vi "FPGA_main_IOtest_v2.vi"() -> ()   [LabVIEW 2020]
doc: "AI and AO only for the required channels, named"
uses:
  Components/FPGA TypeDefs/SelectExcitation_Enum.ctl
  Components/FPGA TypeDefs/SelectAOchannel_Enum.ctl
  <vilib>/Platform/TimedLoop/XDataNode/timing_clust.ctl
  <vilib>/Platform/TimedLoop/XDataNode/nitl_modes.ctl
  <vilib>/Platform/TimedLoop/XDataNode/wakeup.ctl
  <vilib>/rvi/Emulation/niFpgaGetClockAttributes.vi
  <vilib>/rvi/Emulation/niFpgaSctlEmulationGetInTimedLoop.vi
  <vilib>/rvi/Emulation/niFpgaEmulationReportErrorSimple.vi
  <vilib>/rvi/eio/common/nirviEmuTemplateMethod_errors.vi
  <vilib>/rvi/Emulation/niFpgaEmulationIsFPGAContextNoSignature.vi
  <vilib>/rvi/errors/niFpgaSetErrorForExecOnDevCompSimple.vi
  <vilib>/rvi/eio/common/nirviEmuReportErrorAndStop.vi
  <vilib>/rvi/DataTransferAndStorage/Container/Common/niFpgaContainerGetUniqueNameForEmu.vi
  <vilib>/rvi/FIFO/Fifo_Resource/nirvififoEmulationSetSize.vi
  <vilib>/rvi/FIFO/Fifo_Resource/nirviFifoEmulationQueueMgr.vi
  <instcachedir>/0/nirviFifoEmulationQueueMgr_E5CAEC123FF24DC58D834DCA3CDAA9B5.lvgen/nirviFifoEmulationQueueMgr_E5CAEC123FF24DC58D834DCA3CDAA9B5_001.vi
  <vilib>/rvi/FIFO/Fifo_Resource/nirvififoEmulationDetermineInputValidOut.vi
  <vilib>/rvi/FIFO/Fifo_Resource/nirvififoEmulationCreateLock.vi
  <vilib>/rvi/Emulation/niFpgaProcessEmulError.vi
  <vilib>/rvi/FIFO/Fifo_Resource/nirvififoEmulationObtainLock.vi
  <vilib>/rvi/FIFO/Fifo_Resource/nirvififoEmulationReleaseLock.vi
  <vilib>/rvi/occurrence/nirviWaitOnOccurrenceBase.vi
  <vilib>/rvi/errors/nirviReportUnexpectedCaseInternalError.vi
  <vilib>/rvi/errors/nirviReportUnexpectedCaseInternalError (U32).vi
  <vilib>/rvi/Emulation/niFpgaCriticalErrorInLSC.vi
  <vilib>/Utility/error.llb/Clear Errors.vi
  <vilib>/eio/EIONode/EIONode.xnode
  <vilib>/rvi/DataTransferAndStorage/Container/XNode/niFpgaContainer.xnode
  <vilib>/rvi/FIFO/Fifo_Resource/nirvififoEmulationWrite.vi
  <vilib>/rvi/FIFO/Fifo_Resource/nirvififoEmulationRead.vi
  <vilib>/Platform/TimedLoop/XDataNode/XDataNode.xnode
  <vilib>/rvi/FXPMathLib/FxpMul/XNode/nifxpmath_Multiplier.xnode
  Components/FPGA functions/FPGA functions.lvlib
  <vilib>/rvi/FXPMathLib/sim/FxpSim.dll
  <vilib>/Platform/TimedLoop/XDataNode/XDNodeRunTimeDep.lvlib
panel:
  in  "Select AO channel":T1
  out "AO Loop time [ticks]":u32
  in  "Frequency [periods/tick]":fxp<+,32,0>
  in  "Amplitude [V]":fxp<+/-,16,5>
  in  "Excitation mode":T2
  out "AI LS Loop time [ticks]":u32
  out "FPGA AI LS FIFO\nOverflow? 2":bool
  out "AI LS filter Loop time [ticks]":u32
  out "Mod6 (NI 9222) AI":fxp<+/-,25,5>[](array[numeric])
  out "AI LS filter Loop time [ticks]":u32
  out "Mod7 (NI 9222) AI":fxp<+/-,25,5>[](array[numeric])
  out "AI LS Loop time [ticks]":u32
  out "FPGA AI LS FIFO\nOverflow?":bool
  out "Mod8 (NI 9222) AI":fxp<+/-,25,5>[](array[numeric])
  out "AI HS filter Loop time [ticks]":u32
  out "FPGA AI HS FIFO\nOverflow?":bool
  out "AI HS Loop time [ticks]":u32
  # "1 tick = 25 ns"
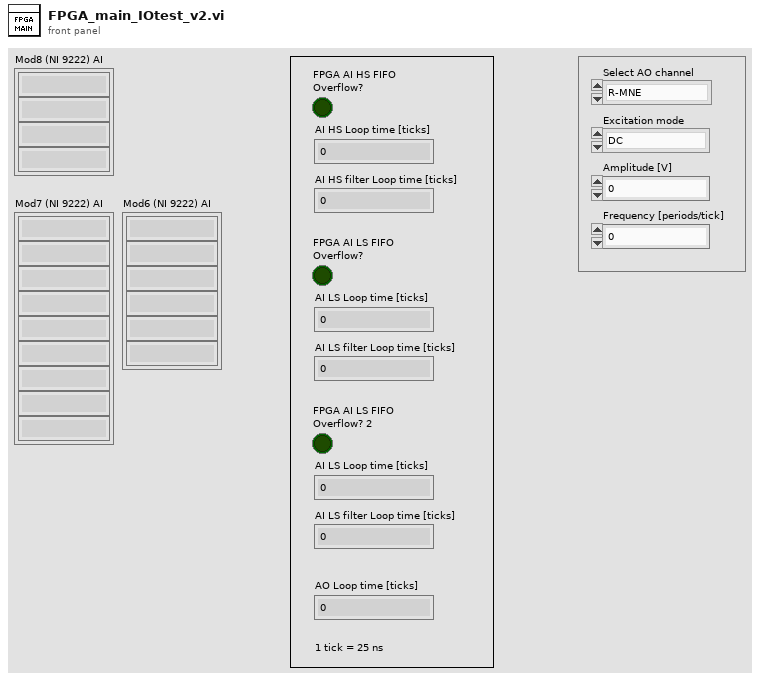
[diagram p1: front panel]
types:
  T1 = typedef "SelectAOchannel_Enum.ctl" = enum16{"R-MNE", "R-MSE", "R-MSW", "R-MNW", "R-CO", "R-CI"}
  T2 = typedef "SelectExcitation_Enum.ctl" = enum16{"DC", "Sinewave", "Squarewave", "WhiteNoise"}
  T3 = typedef "XDNodeRunTimeDep.lvlib/timing_clust.ctl" = cluster{"Expected End [f-1]":u64, "Actual End [f-1]":u64, "Finished Late? [f-1]":bool, "Expected End [i-1]":u64, "Actual End [i-1]":u64, "Finished Late? [i-1]":bool, "Expected Start [i]":u64, "Actual Start [i]":u64, "Expected Start [f]":u64, "Actual Start [f]":u64, "Source Name":string, "Structure Name":string, "Period":i64, "Deadline":i64, "Offset":i64, "Start":i64, "Priority":i32, "Timeout":i32, "Mode":T4, "Wakeup Reason":T5, "Error":errorcluster, "Source Type":string, "Secondary Source Type":string, "Global End Time":u64, "Global Start Time":u64, "Frame Duration":u64, "Iteration Duration":u64, "Assigned CPU":i32, "I/O Scan Engine Mode":u32}
  T4 = typedef "XDNodeRunTimeDep.lvlib/nitl_modes.ctl" = enum32{"No Change", "Process missed periods, maintain original phase", "Discard missed periods, maintain original phase", "Process missed periods, ignore original phase", "Discard missed periods, ignore original phase"}
  T5 = typedef "XDNodeRunTimeDep.lvlib/wakeup.ctl" = enum32{"Normal", "Aborted", "Asynchronous wakeup", "Timing source error", "Timed loop error", "Timeout"}
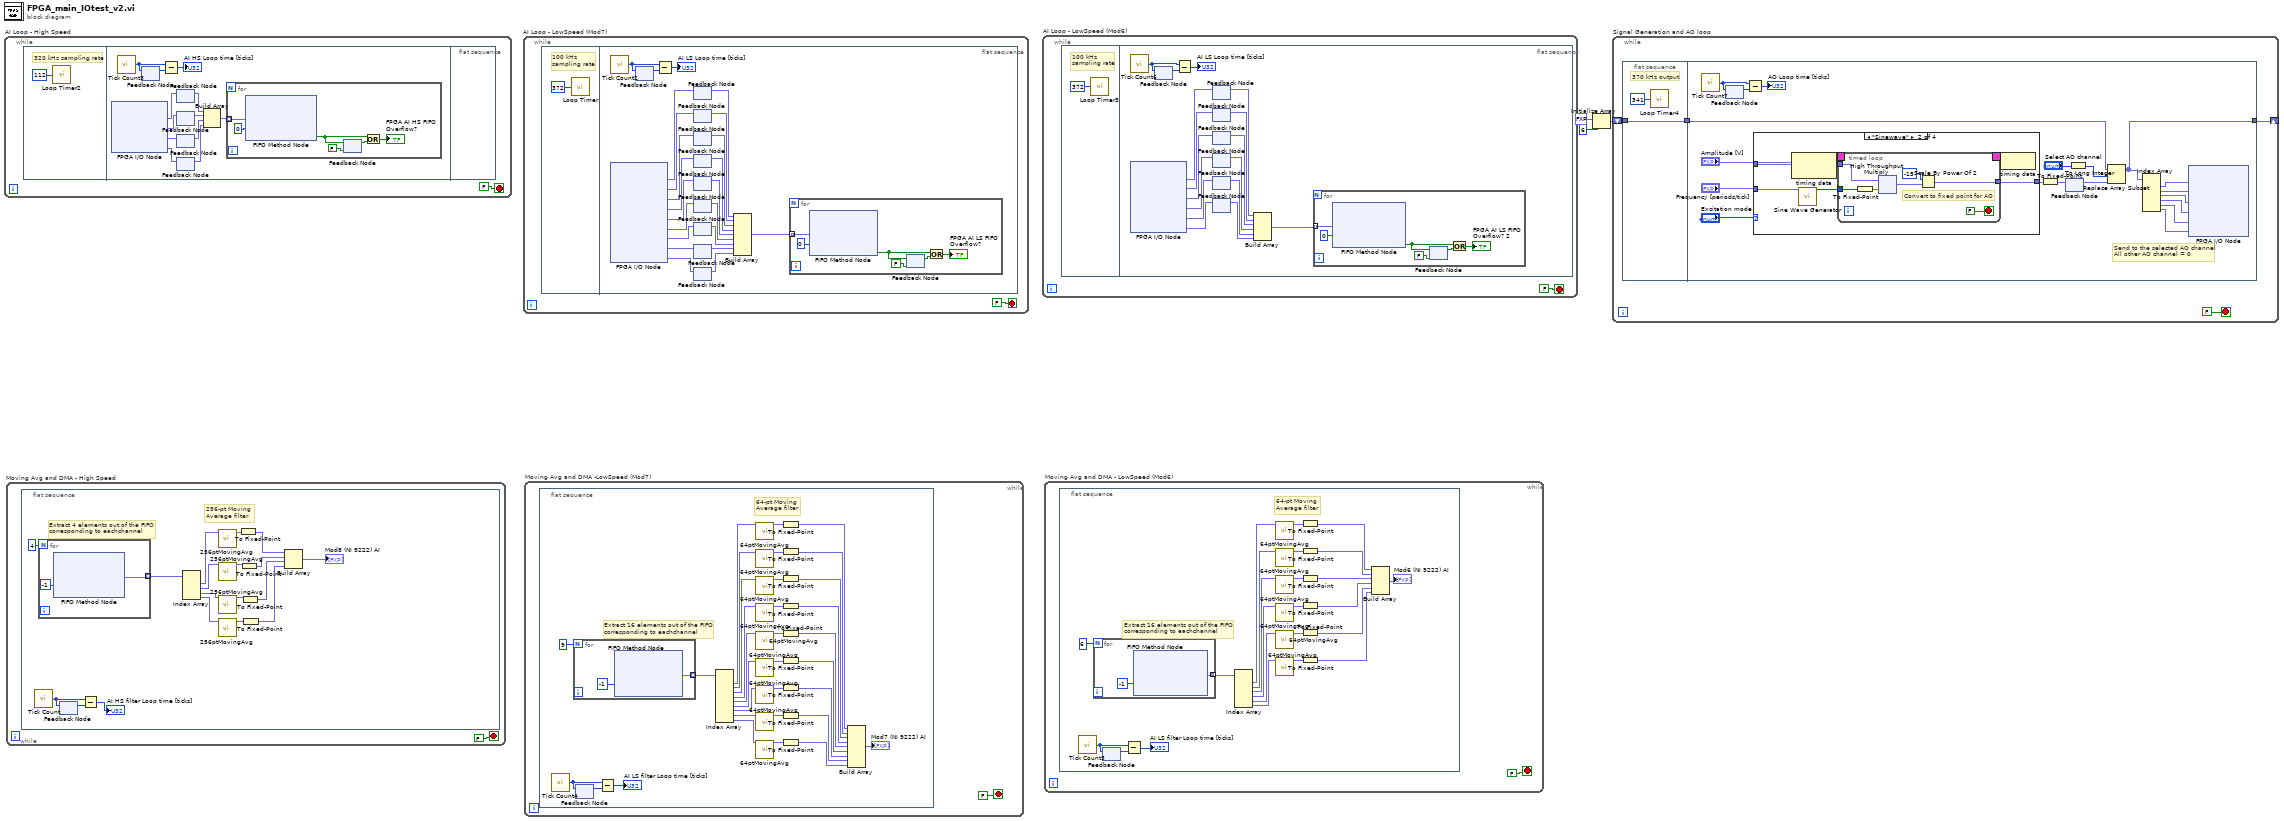
[diagram p0: block diagram]
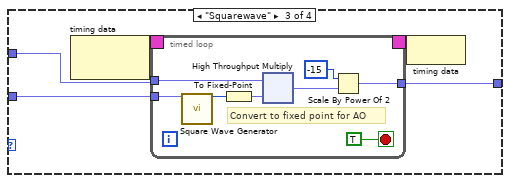
[diagram p3: hidden frame]
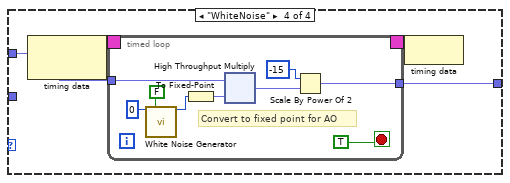
[diagram p4: hidden frame]
diagram:
  n1 = while "AI Loop - High Speed" {
    stop <- FALSE stop-if-true
    n2 = flat-sequence {
      frame #0 {
        # "320 kHz sampling rate"
        n3 = call "Loop Timer2"("Count(Ticks)"=u32 112) -> ()  [unwired: 1 out]
      }
      frame #1 {
        n4 = xnode "FPGA I/O Node"() -> ("Mod8/AI0"=w12:fxp<+/-,24,5>, "Mod8/AI1"=w11:fxp<+/-,24,5>, "Mod8/AI2"=w10:fxp<+/-,24,5>, "Mod8/AI3"=w9:fxp<+/-,24,5>)  [unwired: 4 in, 4 out]
        n5 = call "Tick Count3"() -> ("Tick Count(Ticks)"=w17:u32)
        n6 = feedback #1() -> (w16:u32)  [unwired: 1 in]
        n7 = feedback-in #1(w17) -> ()
        n8 = Subtract(x=w17, y=w16) -> (x-y=→"AI HS Loop time [ticks]":u32)
        n9 = feedback-in #2(w12) -> ()
        n10 = feedback #2() -> (w13:fxp<+/-,24,5>)  [unwired: 1 in]
        n11 = feedback #3() -> (w8:fxp<+/-,24,5>)  [unwired: 1 in]
        n12 = feedback-in #3(w11) -> ()
        n13 = feedback #4() -> (w7:fxp<+/-,24,5>)  [unwired: 1 in]
        n14 = feedback-in #4(w10) -> ()
        n15 = feedback #5() -> (w6:fxp<+/-,24,5>)  [unwired: 1 in]
        n16 = feedback-in #5(w9) -> ()
        n17 = Build Array(w13, w8, w7, w6) -> (w14:fxp<+/-,24,5>[])
        n18 = for {
          tunnel: w14 -> [w22] mode=indexing
          n19 = xnode ("FIFO Method Node")("Element"=w22, "Timeout"=0) -> ("Timed Out?"=w19:bool)  [unwired: 1 in, 1 out]
          n20 = feedback-in #6(w19) -> ()
          n21 = feedback #6(FALSE ("Timed Out?")) -> (w20:bool)
          n22 = Or(x=w19, y=w20) -> (x .or. y?=→"FPGA AI HS FIFO\nOverflow?":bool)
        }
      }
      frame #2 {
      }
    }
  }
  n23 = while "Moving Avg and DMA - High Speed" {
    stop <- FALSE stop-if-true
    n24 = flat-sequence {
      frame #0 {
        # "256-pt Moving \nAverage filter"
        # "Extract 4 elements out of the FIFO \ncorresponding to eachchannel"
        n25 = call "Tick Count"() -> ("Tick Count(Ticks)"=w41:u32)
        n26 = for {
          N: 4 -> [_]
          tunnel: [w43] -> w38 mode=indexing
          n27 = xnode ("FIFO Method Node")("Timeout"=-1) -> ("Element"=w43:fxp<+/-,24,5>)  [unwired: 1 in, 2 out]
        }
        n28 = feedback #7() -> (w40:u32)  [unwired: 1 in]
        n29 = feedback-in #7(w41) -> ()
        n30 = Subtract(x=w41, y=w40) -> (x-y=→"AI HS filter Loop time [ticks]":u32)
        n31 = Index Array(array=w38) -> (element #1=w37:fxp<+/-,24,5>, element #2=w36:fxp<+/-,24,5>, element #3=w34:fxp<+/-,24,5>, element #4=w35:fxp<+/-,24,5>)  [unwired: 4 in]
        n32 = call "256ptMovingAvg.vi"("Raw input"=w37) -> ("Output"=w33:fxp<+/-,28,5>)  [unwired: 10 in]
        n33 = call "256ptMovingAvg.vi"("Raw input"=w36) -> ("Output"=w31:fxp<+/-,28,5>)  [unwired: 10 in]
        n34 = call "256ptMovingAvg.vi"("Raw input"=w34) -> ("Output"=w30:fxp<+/-,28,5>)  [unwired: 10 in]
        n35 = call "256ptMovingAvg.vi"("Raw input"=w35) -> ("Output"=w27:fxp<+/-,28,5>)  [unwired: 10 in]
        n36 = To Fixed-Point(number=w33) -> (fixed-point=w32:fxp<+/-,25,5>)  [unwired: 1 in]
        n37 = To Fixed-Point(number=w31) -> (fixed-point=w29:fxp<+/-,25,5>)  [unwired: 1 in]
        n38 = To Fixed-Point(number=w30) -> (fixed-point=w28:fxp<+/-,25,5>)  [unwired: 1 in]
        n39 = To Fixed-Point(number=w27) -> (fixed-point=w26:fxp<+/-,25,5>)  [unwired: 1 in]
        n40 = Build Array(w32, w29, w28, w26) -> (→"Mod8 (NI 9222) AI":fxp<+/-,25,5>[])
      }
    }
  }
  n41 = while "AI Loop - LowSpeed (Mod7)" {
    stop <- FALSE stop-if-true
    n42 = flat-sequence {
      frame #0 {
        # "100 kHz \nsampling rate"
        n43 = call "Loop Timer"("Count(Ticks)"=u32 372) -> ()  [unwired: 1 out]
      }
      frame #1 {
        n44 = call "Tick Count2"() -> ("Tick Count(Ticks)"=w68:u32)
        n45 = xnode "FPGA I/O Node"() -> ("Mod7/AI0"=w64:fxp<+/-,24,5>, "Mod7/AI1"=w63:fxp<+/-,24,5>, "Mod7/AI2"=w62:fxp<+/-,24,5>, "Mod7/AI3"=w61:fxp<+/-,24,5>, "Mod7/AI4"=w60:fxp<+/-,24,5>, "Mod7/AI5"=w59:fxp<+/-,24,5>, "Mod7/AI6"=w58:fxp<+/-,24,5>, "Mod7/AI7"=w57:fxp<+/-,24,5>, "Mod7/AI8"=w56:fxp<+/-,24,5>)  [unwired: 9 in, 9 out]
        n46 = feedback #8() -> (w67:u32)  [unwired: 1 in]
        n47 = feedback-in #8(w68) -> ()
        n48 = Subtract(x=w68, y=w67) -> (x-y=→"AI LS Loop time [ticks]":u32)
        n49 = feedback #9() -> (w55:fxp<+/-,24,5>)  [unwired: 1 in]
        n50 = feedback-in #9(w64) -> ()
        n51 = feedback #10() -> (w54:fxp<+/-,24,5>)  [unwired: 1 in]
        n52 = feedback-in #10(w63) -> ()
        n53 = feedback #11() -> (w53:fxp<+/-,24,5>)  [unwired: 1 in]
        n54 = feedback-in #11(w62) -> ()
        n55 = feedback #12() -> (w52:fxp<+/-,24,5>)  [unwired: 1 in]
        n56 = feedback-in #12(w61) -> ()
        n57 = feedback #13() -> (w51:fxp<+/-,24,5>)  [unwired: 1 in]
        n58 = feedback-in #13(w60) -> ()
        n59 = feedback #14() -> (w50:fxp<+/-,24,5>)  [unwired: 1 in]
        n60 = feedback-in #14(w59) -> ()
        n61 = feedback #15() -> (w49:fxp<+/-,24,5>)  [unwired: 1 in]
        n62 = feedback-in #15(w58) -> ()
        n63 = feedback #16() -> (w48:fxp<+/-,24,5>)  [unwired: 1 in]
        n64 = feedback-in #16(w57) -> ()
        n65 = feedback #17() -> (w47:fxp<+/-,24,5>)  [unwired: 1 in]
        n66 = feedback-in #17(w56) -> ()
        n67 = Build Array(w55, w54, w53, w52, w51, w50, w49, w48, w47) -> (w65:fxp<+/-,24,5>[])
        n68 = for {
          tunnel: w65 -> [w69] mode=indexing
          n69 = xnode ("FIFO Method Node")("Element"=w69, "Timeout"=0) -> ("Timed Out?"=w71:bool)  [unwired: 1 in, 1 out]
          n70 = feedback-in #18(w71) -> ()
          n71 = feedback #18(FALSE ("Timed Out?")) -> (w72:bool)
          n72 = Or(x=w71, y=w72) -> (x .or. y?=→"FPGA AI LS FIFO\nOverflow?":bool)
        }
      }
    }
  }
  n73 = while "Moving Avg and DMA -LowSpeed (Mod7)" {
    stop <- FALSE stop-if-true
    n74 = flat-sequence {
      frame #0 {
        # "64-pt Moving \nAverage filter"
        # "Extract 16 elements out of the FIFO \ncorresponding to eachchannel"
        n75 = call "Tick Count4"() -> ("Tick Count(Ticks)"=w107:u32)
        n76 = for {
          N: 9 -> [_]
          tunnel: [w109] -> w104 mode=indexing
          n77 = xnode ("FIFO Method Node")("Timeout"=-1) -> ("Element"=w109:fxp<+/-,24,5>)  [unwired: 1 in, 2 out]
        }
        n78 = feedback #19() -> (w106:u32)  [unwired: 1 in]
        n79 = feedback-in #19(w107) -> ()
        n80 = Subtract(x=w107, y=w106) -> (x-y=→"AI LS filter Loop time [ticks]":u32)
        n81 = Index Array(array=w104) -> (element #1=w101:fxp<+/-,24,5>, element #2=w100:fxp<+/-,24,5>, element #3=w99:fxp<+/-,24,5>, element #4=w98:fxp<+/-,24,5>, element #5=w97:fxp<+/-,24,5>, element #6=w96:fxp<+/-,24,5>, element #7=w95:fxp<+/-,24,5>, element #8=w94:fxp<+/-,24,5>, element #9=w93:fxp<+/-,24,5>)  [unwired: 9 in]
        n82 = call "64ptMovingAvg.vi"("Raw input"=w101) -> ("Output"=w92:fxp<+/-,28,5>)  [unwired: 10 in]
        n83 = call "64ptMovingAvg.vi"("Raw input"=w100) -> ("Output"=w91:fxp<+/-,28,5>)  [unwired: 10 in]
        n84 = call "64ptMovingAvg.vi"("Raw input"=w99) -> ("Output"=w90:fxp<+/-,28,5>)  [unwired: 10 in]
        n85 = call "64ptMovingAvg.vi"("Raw input"=w98) -> ("Output"=w89:fxp<+/-,28,5>)  [unwired: 10 in]
        n86 = call "64ptMovingAvg.vi"("Raw input"=w97) -> ("Output"=w88:fxp<+/-,28,5>)  [unwired: 10 in]
        n87 = call "64ptMovingAvg.vi"("Raw input"=w96) -> ("Output"=w87:fxp<+/-,28,5>)  [unwired: 10 in]
        n88 = call "64ptMovingAvg.vi"("Raw input"=w95) -> ("Output"=w86:fxp<+/-,28,5>)  [unwired: 10 in]
        n89 = call "64ptMovingAvg.vi"("Raw input"=w94) -> ("Output"=w85:fxp<+/-,28,5>)  [unwired: 10 in]
        n90 = call "64ptMovingAvg.vi"("Raw input"=w93) -> ("Output"=w84:fxp<+/-,28,5>)  [unwired: 10 in]
        n91 = To Fixed-Point(number=w92) -> (fixed-point=w103:fxp<+/-,25,5>)  [unwired: 1 in]
        n92 = To Fixed-Point(number=w91) -> (fixed-point=w83:fxp<+/-,25,5>)  [unwired: 1 in]
        n93 = To Fixed-Point(number=w90) -> (fixed-point=w82:fxp<+/-,25,5>)  [unwired: 1 in]
        n94 = To Fixed-Point(number=w89) -> (fixed-point=w81:fxp<+/-,25,5>)  [unwired: 1 in]
        n95 = To Fixed-Point(number=w88) -> (fixed-point=w80:fxp<+/-,25,5>)  [unwired: 1 in]
        n96 = To Fixed-Point(number=w87) -> (fixed-point=w79:fxp<+/-,25,5>)  [unwired: 1 in]
        n97 = To Fixed-Point(number=w86) -> (fixed-point=w78:fxp<+/-,25,5>)  [unwired: 1 in]
        n98 = To Fixed-Point(number=w85) -> (fixed-point=w77:fxp<+/-,25,5>)  [unwired: 1 in]
        n99 = To Fixed-Point(number=w84) -> (fixed-point=w76:fxp<+/-,25,5>)  [unwired: 1 in]
        n100 = Build Array(w103, w83, w82, w81, w80, w79, w78, w77, w76) -> (→"Mod7 (NI 9222) AI":fxp<+/-,25,5>[])
      }
    }
  }
  n101 = while "AI Loop - LowSpeed (Mod6)" {
    stop <- FALSE stop-if-true
    n102 = flat-sequence {
      frame #0 {
        # "100 kHz \nsampling rate"
        n103 = call "Loop Timer3"("Count(Ticks)"=u32 372) -> ()  [unwired: 1 out]
      }
      frame #1 {
        n104 = call "Tick Count6"() -> ("Tick Count(Ticks)"=w128:u32)
        n105 = xnode "FPGA I/O Node"() -> ("Mod6/AI0"=w124:fxp<+/-,24,5>, "Mod6/AI1"=w117:fxp<+/-,24,5>, "Mod6/AI2"=w116:fxp<+/-,24,5>, "Mod6/AI3"=w115:fxp<+/-,24,5>, "Mod6/AI4"=w114:fxp<+/-,24,5>, "Mod6/AI5"=w113:fxp<+/-,24,5>)  [unwired: 6 in, 6 out]
        n106 = feedback #20() -> (w127:u32)  [unwired: 1 in]
        n107 = feedback-in #20(w128) -> ()
        n108 = Subtract(x=w128, y=w127) -> (x-y=→"AI LS Loop time [ticks]":u32)
        n109 = feedback #21() -> (w123:fxp<+/-,24,5>)  [unwired: 1 in]
        n110 = feedback-in #21(w124) -> ()
        n111 = feedback #22() -> (w122:fxp<+/-,24,5>)  [unwired: 1 in]
        n112 = feedback-in #22(w117) -> ()
        n113 = feedback #23() -> (w121:fxp<+/-,24,5>)  [unwired: 1 in]
        n114 = feedback-in #23(w116) -> ()
        n115 = feedback #24() -> (w120:fxp<+/-,24,5>)  [unwired: 1 in]
        n116 = feedback-in #24(w115) -> ()
        n117 = feedback #25() -> (w119:fxp<+/-,24,5>)  [unwired: 1 in]
        n118 = feedback-in #25(w114) -> ()
        n119 = feedback #26() -> (w118:fxp<+/-,24,5>)  [unwired: 1 in]
        n120 = feedback-in #26(w113) -> ()
        n121 = Build Array(w123, w122, w121, w120, w119, w118) -> (w125:fxp<+/-,24,5>[])
        n122 = for {
          tunnel: w125 -> [w129] mode=indexing
          n123 = xnode ("FIFO Method Node")("Element"=w129, "Timeout"=0) -> ("Timed Out?"=w131:bool)  [unwired: 1 in, 1 out]
          n124 = feedback-in #27(w131) -> ()
          n125 = feedback #27(FALSE ("Timed Out?")) -> (w132:bool)
          n126 = Or(x=w131, y=w132) -> (x .or. y?=→"FPGA AI LS FIFO\nOverflow? 2":bool)
        }
      }
    }
  }
  n127 = while "Moving Avg and DMA - LowSpeed (Mod6)" {
    stop <- FALSE stop-if-true
    n128 = flat-sequence {
      frame #0 {
        # "64-pt Moving \nAverage filter"
        # "Extract 16 elements out of the FIFO \ncorresponding to eachchannel"
        n129 = call "Tick Count5"() -> ("Tick Count(Ticks)"=w158:u32)
        n130 = for {
          N: 6 -> [_]
          tunnel: [w160] -> w155 mode=indexing
          n131 = xnode ("FIFO Method Node")("Timeout"=-1) -> ("Element"=w160:fxp<+/-,24,5>)  [unwired: 1 in, 2 out]
        }
        n132 = feedback #28() -> (w157:u32)  [unwired: 1 in]
        n133 = feedback-in #28(w158) -> ()
        n134 = Subtract(x=w158, y=w157) -> (x-y=→"AI LS filter Loop time [ticks]":u32)
        n135 = Index Array(array=w155) -> (element #1=w153:fxp<+/-,24,5>, element #2=w152:fxp<+/-,24,5>, element #3=w151:fxp<+/-,24,5>, element #4=w150:fxp<+/-,24,5>, element #5=w149:fxp<+/-,24,5>, element #6=w148:fxp<+/-,24,5>)  [unwired: 6 in]
        n136 = call "64ptMovingAvg.vi"("Raw input"=w153) -> ("Output"=w147:fxp<+/-,28,5>)  [unwired: 10 in]
        n137 = call "64ptMovingAvg.vi"("Raw input"=w152) -> ("Output"=w146:fxp<+/-,28,5>)  [unwired: 10 in]
        n138 = call "64ptMovingAvg.vi"("Raw input"=w151) -> ("Output"=w145:fxp<+/-,28,5>)  [unwired: 10 in]
        n139 = call "64ptMovingAvg.vi"("Raw input"=w150) -> ("Output"=w144:fxp<+/-,28,5>)  [unwired: 10 in]
        n140 = call "64ptMovingAvg.vi"("Raw input"=w149) -> ("Output"=w143:fxp<+/-,28,5>)  [unwired: 10 in]
        n141 = call "64ptMovingAvg.vi"("Raw input"=w148) -> ("Output"=w142:fxp<+/-,28,5>)  [unwired: 10 in]
        n142 = To Fixed-Point(number=w147) -> (fixed-point=w154:fxp<+/-,25,5>)  [unwired: 1 in]
        n143 = To Fixed-Point(number=w146) -> (fixed-point=w141:fxp<+/-,25,5>)  [unwired: 1 in]
        n144 = To Fixed-Point(number=w145) -> (fixed-point=w140:fxp<+/-,25,5>)  [unwired: 1 in]
        n145 = To Fixed-Point(number=w144) -> (fixed-point=w139:fxp<+/-,25,5>)  [unwired: 1 in]
        n146 = To Fixed-Point(number=w143) -> (fixed-point=w138:fxp<+/-,25,5>)  [unwired: 1 in]
        n147 = To Fixed-Point(number=w142) -> (fixed-point=w137:fxp<+/-,25,5>)  [unwired: 1 in]
        n148 = Build Array(w154, w141, w140, w139, w138, w137) -> (→"Mod6 (NI 9222) AI":fxp<+/-,25,5>[])
      }
    }
  }
  n149 = Initialize Array(fxp<+/-,20,5> 0.0 ("element"), 6 ("dimension size")) -> (w3:fxp<+/-,20,5>[])
  n150 = while "Signal Generation and AO loop" {
    shift-right: [w164] -> _
    shift-left: w3 -> [w163]
    stop <- FALSE stop-if-true
    n151 = flat-sequence {
      tunnel: w163 -> [w166]
      tunnel: [w166] -> w162
      tunnel: [w173] -> w164
      tunnel: w162 -> [w178]
      frame #0 {
        # "370 kHz output"
        n152 = call "Loop Timer4"("Count(Ticks)"=u32 341) -> ()  [unwired: 1 out]
      }
      frame #1 {
        # "Send to the selected AO channel\nAll other AO channel = 0"
        n153 = call "Tick Count7"() -> ("Tick Count(Ticks)"=w182:u32)
        n154 = feedback #29() -> (w181:u32)  [unwired: 1 in]
        n155 = feedback-in #29(w182) -> ()
        n156 = Subtract(x=w182, y=w181) -> (x-y=→"AO Loop time [ticks]":u32)
        n157 = case shown="\"Sinewave\"" "Excitation mode" {
          tunnel: "Amplitude [V]" -> [w187 w192 w208 w225]
          tunnel: [w187 w191 w207 w224] -> w183
          tunnel: "Frequency [periods/tick]" -> [_ w190 w209 _]
          frame "DC", Default {
          }
          frame "Sinewave" {
            n158 = node-c288() -> (w189:T3)  [unwired: 1 in]
            n159 = call "Sine Wave Generator"("frequency (periods/tick)"=w190) -> ("sine out"=w193:i16)  [unwired: 14 in]
            n160 = timed-loop {
              timing: w189 -> [_]
              timing-out: [_] -> w188
              tunnel: w193 -> [w199]
              tunnel: w192 -> [w198]
              tunnel: [w195] -> w191
              stop <- FALSE stop-if-true
              # "Convert to fixed point for AO"
              n161 = To Fixed-Point(number=w199) -> (fixed-point=w200:fxp<+/-,16,16>)  [unwired: 1 in]
              n162 = xnode ("High Throughput Multiply")("x"=w198, "y"=w200) -> ("x*y"=w197:fxp<+/-,32,21>)
              n163 = Scale By Power Of 2(n=i16 -15, x=w197) -> (x*2^n=w195:fxp<+/-,32,21>)
            }
            n164 = node-c288(w188) -> ()
          }
          frame "Squarewave" {
            n165 = node-c288() -> (w206:T3)  [unwired: 1 in]
            n166 = timed-loop {
              timing: w206 -> [_]
              timing-out: [_] -> w205
              tunnel: w209 -> [w217]
              tunnel: w208 -> [w212]
              tunnel: [w211] -> w207
              stop <- TRUE stop-if-true
              # "Convert to fixed point for AO"
              n167 = call "Square Wave Generator"("frequency (periods/tick)"=w217) -> ("square wave out"=w213:i16)  [unwired: 14 in]
              n168 = To Fixed-Point(number=w213) -> (fixed-point=w216:fxp<+/-,16,16>)  [unwired: 1 in]
              n169 = xnode ("High Throughput Multiply")("x"=w212, "y"=w216) -> ("x*y"=w215:fxp<+/-,32,21>)
              n170 = Scale By Power Of 2(n=i16 -15, x=w215) -> (x*2^n=w211:fxp<+/-,32,21>)
            }
            n171 = node-c288(w205) -> ()
          }
          frame "WhiteNoise" {
            n172 = node-c288() -> (w223:T3)  [unwired: 1 in]
            n173 = timed-loop {
              timing: w223 -> [_]
              timing-out: [_] -> w222
              tunnel: w225 -> [w230]
              tunnel: [w229] -> w224
              stop <- TRUE stop-if-true
              # "Convert to fixed point for AO"
              n174 = call "White Noise Generator"("seed"=u32 0, "reset"=FALSE) -> ("white noise out"=w231:i16)  [unwired: 13 in]
              n175 = To Fixed-Point(number=w231) -> (fixed-point=w234:fxp<+/-,16,16>)  [unwired: 1 in]
              n176 = xnode ("High Throughput Multiply")("x"=w230, "y"=w234) -> ("x*y"=w233:fxp<+/-,32,21>)
              n177 = Scale By Power Of 2(n=i16 -15, x=w233) -> (x*2^n=w229:fxp<+/-,32,21>)
            }
            n178 = node-c288(w222) -> ()
          }
        }
        n179 = To Fixed-Point(number=w183) -> (fixed-point=w179:fxp<+/-,20,5>)  [unwired: 1 in]
        n180 = feedback #30() -> (w175:fxp<+/-,20,5>)  [unwired: 1 in]
        n181 = feedback-in #30(w179) -> ()
        n182 = To Long Integer(number="Select AO channel") -> (32bit integer=w177:i32)
        n183 = Replace Array Subset(array=w178, new element=w175, index=w177) -> (w173:fxp<+/-,20,5>[])
        n184 = Index Array(array=w173) -> (element #1=w174:fxp<+/-,20,5>, element #2=w172:fxp<+/-,20,5>, element #3=w171:fxp<+/-,20,5>, element #4=w170:fxp<+/-,20,5>, element #5=w169:fxp<+/-,20,5>, element #6=w168:fxp<+/-,20,5>)  [unwired: 6 in]
        n185 = xnode "FPGA I/O Node"("Mod3/AO0"=w174, "Mod3/AO1"=w172, "Mod3/AO2"=w171, "Mod3/AO3"=w170, "Mod4/AO0"=w169, "Mod4/AO1"=w168) -> ()  [unwired: 6 in, 6 out]
      }
    }
  }
